vi "VD-freeRunRead.vi"(8 "error in (no error)":errorcluster, 11 "VD-LV-LiteVNA in":refnum<class "VD-LV-LiteVNA.lvclass">) -> (0 "error out":errorcluster, 3 "VD-LV-LiteVNA out":refnum<class "VD-LV-LiteVNA.lvclass">)   [LabVIEW 2020, in "VD-LV-LiteVNA.lvclass"]
uses:
  VD-LV-LiteVNA.lvclass
  VD-LV-LiteVNA.lvclass/VD-LV-LiteVNA.ctl
  hardware-protocol/serial/HP-S-Serial.lvclass
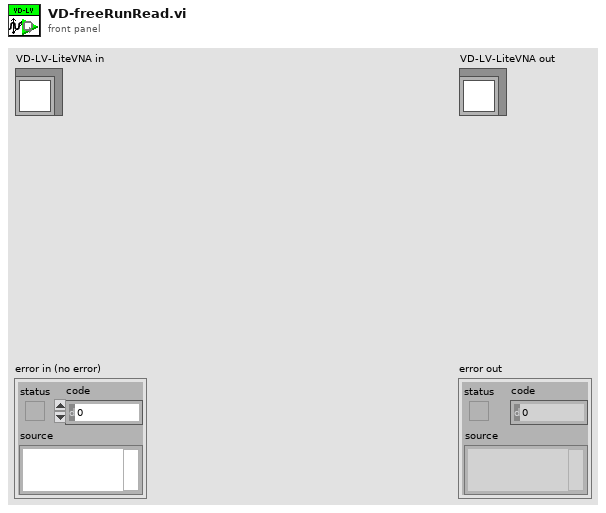
[diagram p1: front panel]
types:
  T1 = typedef "HP-S-Serial.lvclass/HP-S-data.ctl" = u8[]
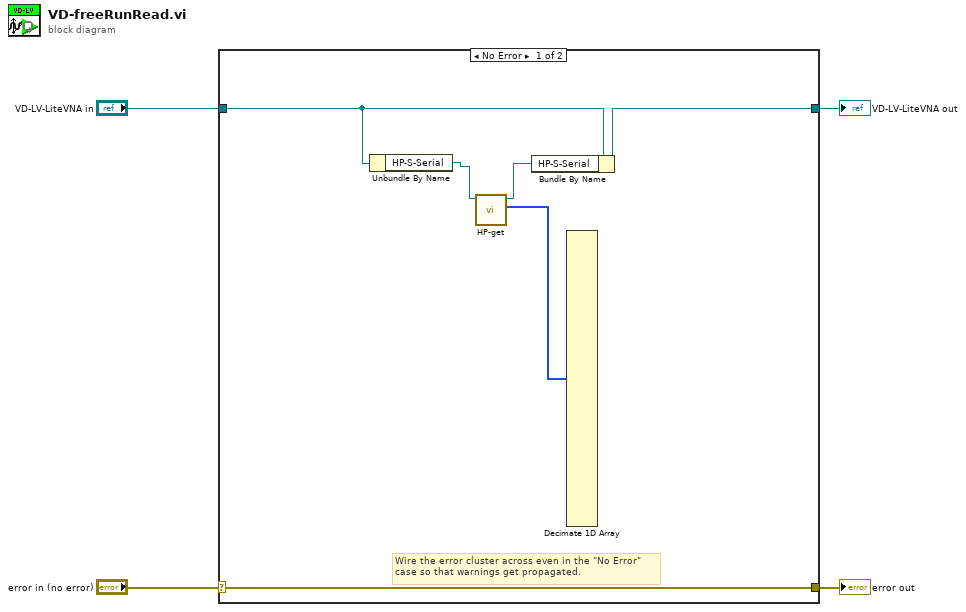
[diagram p0: block diagram]
diagram:
  n1 = case shown="No Error" "error in (no error)" {
    selector: "error in (no error)" -> [w10 w12]
    tunnel: [w10 w12] -> w3
    tunnel: [w6 w11] -> w1
    tunnel: "VD-LV-LiteVNA in" -> [w7 w11]
    frame No Error {
      # "Wire the error cluster across even in the \"No Error\"\ncase so that warnings get propagated."
      n2 = Unbundle By Name(w7) -> ("HP-S-Serial"=w9:refnum<class "HP-S-Serial.lvclass">)
      n3 = call-dynamic "HP-get.vi"("HP-S-Serial in"=w9) -> ("read buffer"=w5:T1, "HP-S-Serial out"=w8:refnum<class "HP-S-Serial.lvclass">)  [unwired: 8 in, 1 out]
      n4 = Bundle By Name(cluster=w7, "HP-S-Serial"=w8) -> (w6:refnum<class "VD-LV-LiteVNA.lvclass">)
      n5 = Decimate 1D Array(w5) -> ()  [unwired: 37 out]
    }
    frame Error {
    }
  }
  "error out" <- w3
  "VD-LV-LiteVNA out" <- w1
